vi "REM IO - Get Slave IOVars.vi"(8 "error in (no error)":errorcluster, 11 "ECAT Slave in":refnum<k21>="ni.var.io://localhost/EtherCAT Master/Device") -> (0 "error IO":errorcluster, 1 "REM IO Modules":refnum<k21>[](array[refnum]), 2 "ECAT Variablenobjekt":refnum<k21>[](array[refnum]), 3 "ECAT Slave out":refnum<k21>="ni.var.io:/")   [LabVIEW 2020, in "SEECD Engine.lvlib"]
uses:
  SEECD Engine.lvlib
  <resource>/objmgr/IndComECAT.rc
  <vilib>/NI VeriStand/Custom Device Tools/Custom Device Utility Library/Custom Device Utility Library.lvlib
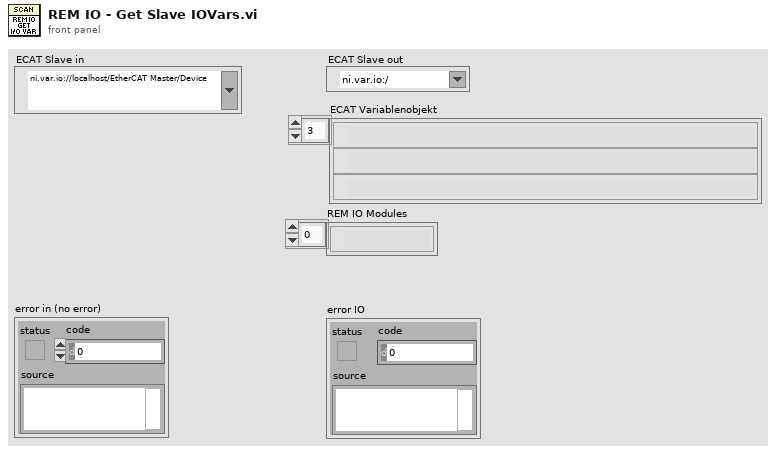
[diagram p1: front panel]
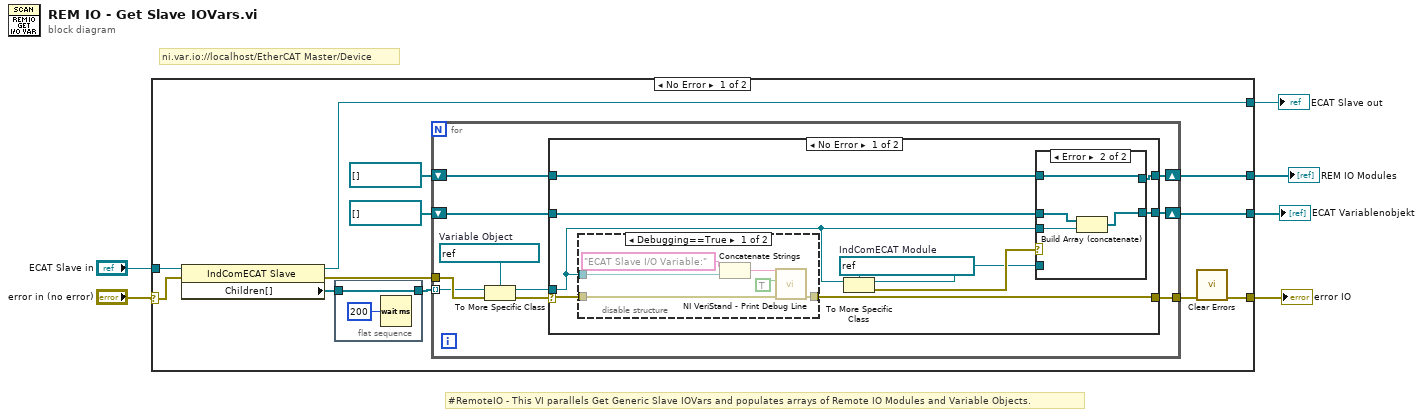
[diagram p0: block diagram]
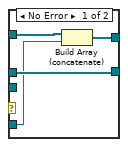
[diagram p3: hidden frame]
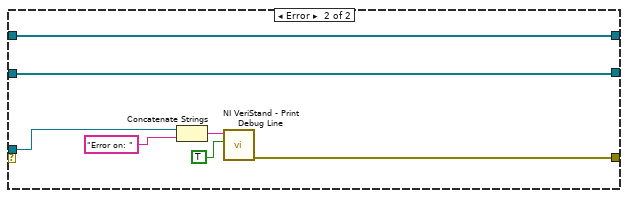
[diagram p4: hidden frame]
diagram:
  # "#RemoteIO - This VI parallels Get Generic Slave IOVars and populates arrays of Remote IO Modules and Variable Objects."
  # "ni.var.io://localhost/EtherCAT Master/Device"
  n1 = case shown="No Error" "error in (no error)" {
    selector: "error in (no error)" -> [w16 w64]
    tunnel: [w7 w64] -> w2
    tunnel: "ECAT Slave in" -> [w18 w63]
    tunnel: [w17 w63] -> w5
    tunnel: [w10 _] -> w3
    tunnel: [w8 _] -> w1
    frame No Error {
      n2 = property class="IndComECAT Slave"(reference=w18, error in=w16) -> (reference out=w17:refnum<k21>, error out=w15:errorcluster, "Children[]"=w13:refnum<k21>[])
      n3 = flat-sequence {
        tunnel: w13 -> [w20]
        tunnel: [w20] -> w12
        frame #0 {
          n4 = Wait (ms)(milliseconds to wait=u32 200) -> ()  [unwired: 1 out]
        }
      }
      n5 = for {
        tunnel: w12 -> [w26] mode=indexing
        tunnel: w15 -> [w30]
        tunnel: [w29] -> w14
        shift-right: [w25] -> w10
        shift-left: refnum<k21>[] [] -> [w24]
        shift-right: [w21] -> w8
        shift-left: refnum<k21>[] [] -> [w22]
        w23 = refnum<k21> refnum  # Variable Object
        n6 = To More Specific Class(target class=w23, reference=w26, error in=w30) -> (specific class reference=w27:refnum<k21>, error out=w28:errorcluster)
        n7 = case shown="No Error" w28 {
          selector: w28 -> [w37 _]
          tunnel: w27 -> [w35 w61]
          tunnel: [w38 w58] -> w29
          tunnel: [w39 w62] -> w25
          tunnel: w24 -> [w40 w62]
          tunnel: w22 -> [w33 w56]
          tunnel: [w32 w56] -> w21
          frame No Error {
            w36 = refnum<k21> refnum  # IndComECAT Module
            n8 = disable-structure shown="Debugging==True" {
              disable-tunnel: [w45 w47] -> w38
              disable-tunnel: w37 -> [w44 w47]
              disable-tunnel: w35 -> [w41 _]
              frame condition #0 {
                n9 = Concatenate Strings("ECAT Slave I/O Variable:", w41) -> (w43:string)
                n10 = call <vilib>:"NI VeriStand - Print Debug Line.vi"("error in (no error)"=w44, "Add to log file? (F)"=TRUE, "Message"=w43) -> ("error out"=w45:errorcluster)  [unwired: 8 in]
              }
              frame condition #1 (active) {
              }
            }
            n11 = To More Specific Class(target class=w36, reference=w35) -> (specific class reference=w31:refnum<k21>, error out=w34:errorcluster)  [unwired: 1 in]
            n12 = case shown="Error" w34 {
              tunnel: w40 -> [w49 w55]
              tunnel: [w49 w53] -> w39
              tunnel: w35 -> [_ w54]
              tunnel: w33 -> [w51 w52]
              tunnel: [w50 w52] -> w32
              tunnel: w31 -> [w48 _]
              frame No Error {
                n13 = Build Array (concatenate)(w51, w48) -> (w50:refnum<k21>[])
              }
              frame Error {
                n14 = Build Array (concatenate)(w55, w54) -> (w53:refnum<k21>[])
              }
            }
          }
          frame Error {
            n15 = Concatenate Strings(w61, "Error on: ") -> (w59:string)
            n16 = call <vilib>:"NI VeriStand - Print Debug Line.vi"("Add to log file? (F)"=TRUE ("Add to log file? (T)"), "Message"=w59) -> ("error out"=w58:errorcluster)  [unwired: 9 in]
          }
        }
      }
      n17 = call <vilib>:"Clear Errors.vi"("error in (no error)"=w14) -> ("error out"=w7:errorcluster)  [unwired: 5 in, 1 out]
    }
    frame Error {
    }
  }
  "error IO" <- w2
  "ECAT Slave out" <- w5
  "ECAT Variablenobjekt" <- w3
  "REM IO Modules" <- w1
